vi "Remove Wall Complete Lines.vi"(8 "entrée d'erreur (pas d'erreur)":errorcluster, 9 "Lines Size List":i32[](array[numeric]), 10 "Brick Wall In":T1[](array[typedef]), 11 "Game Board In":refnum<class "Game Board.lvclass">) -> (0 "sortie d'erreur":errorcluster caption="error out", 1 "Brick Wall Out":T1[](array[typedef]), 3 "Game Board Out":refnum<class "Game Board.lvclass">)   [LabVIEW 2017, in "Game Board.lvclass"]
uses:
  Game Board.lvclass
  Controls/Coordinates.ctl
  Game Board.lvclass/Game Board.ctl
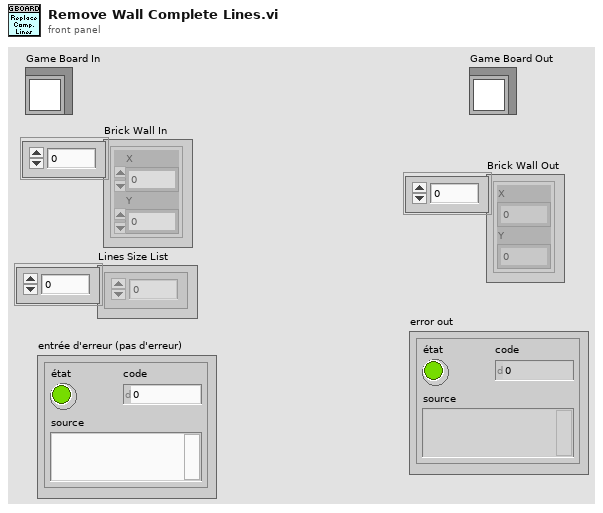
[diagram p1: front panel]
types:
  T1 = typedef "Coordinates.ctl" = cluster{"X":i32, "Y":i32}
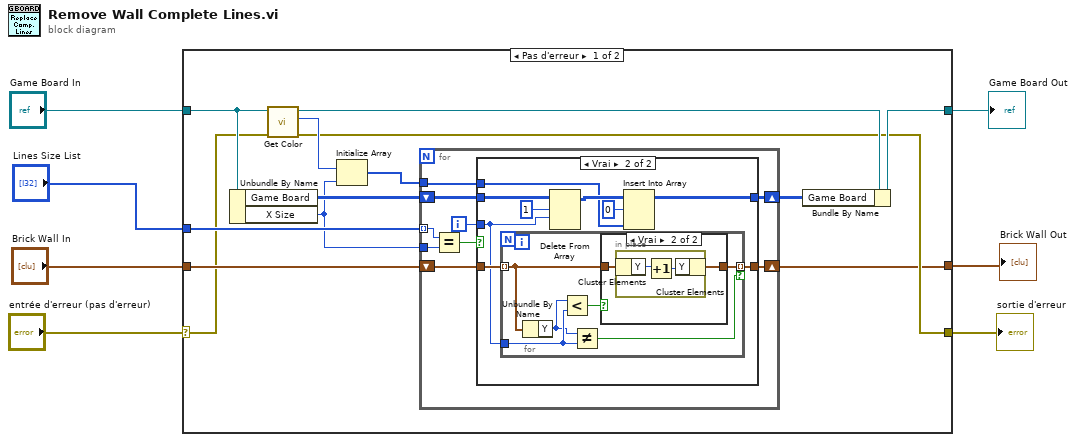
[diagram p0: block diagram]
diagram:
  n1 = case shown="Pas d'erreur" "entrée d'erreur (pas d'erreur)" {
    selector: "entrée d'erreur (pas d'erreur)" -> [w11 w53]
    tunnel: "Game Board In" -> [w12 w54]
    tunnel: [w10 w54] -> w5
    tunnel: [w9 w53] -> w4
    tunnel: "Brick Wall In" -> [w16 w52]
    tunnel: "Lines Size List" -> [w14 _]
    tunnel: [w8 w52] -> w1
    frame No Error {
      n2 = Unbundle By Name(w12) -> ("Game Board"=w17:u32[][], "X Size"=w13:i32)
      n3 = call-dynamic "Get Color.vi"("error in (no error)"=w11, "object in"=w12) -> ("error out"=w9:errorcluster, "Color"=w19:u32, "object out"=w18:refnum<class "Game Board.lvclass">)  [unwired: 7 in]
      n4 = Initialize Array(w19, w13) -> (w20:u32[])
      n5 = for {
        tunnel: w13 -> [w29]
        shift-right: [w27] -> w15
        shift-left: w17 -> [w28]
        tunnel: w20 -> [w24]
        shift-right: [w21] -> w8
        shift-left: w16 -> [w22]
        tunnel: w14 -> [w23] mode=indexing
        i -> [w25]
        n6 = Equal?(x=w23, y=w29) -> (x = y?=w26:bool)
        n7 = case shown="Vrai" w26 {
          tunnel: w28 -> [w31 w40]
          tunnel: [w31 w37] -> w27
          tunnel: w25 -> [_ w33]
          tunnel: w24 -> [_ w36]
          tunnel: w22 -> [w30 w35]
          tunnel: [w30 w34] -> w21
          frame False {
          }
          frame True {
            n8 = for {
              tunnel: w35 -> [w42] mode=indexing
              tunnel: [w41] -> w34 mode=indexing if=w46
              tunnel: w33 -> [w45]
              n9 = Unbundle By Name(w42) -> ("Y"=w44:i32)
              n10 = Less?(x=w44, y=w45) -> (x < y?=w43:bool)
              n11 = Not Equal?(x=w44, y=w45) -> (x != y?=w46:bool)
              n12 = case shown="Vrai" w43 {
                tunnel: w42 -> [w47 w49]
                tunnel: [w47 w48] -> w41
                frame False {
                }
                frame True {
                  n13 = in-place {
                    n14 = in-place-cluster #1(w49) -> ("Y"=w51:i32)
                    n15 = Increment(x=w51) -> (x+1=w50:i32)
                    n16 = in-place-cluster #1("Y"=w50) -> (w48:T1)
                  }
                }
              }
            }
            n17 = Delete From Array(array=w40, length=1 ("longueur"), index (row)=w33) -> (array with subset deleted=w38:u32[][])  [unwired: 1 in, 1 out]
            n18 = Insert Into Array(array=w38, index (row)=0 ("indice (ligne)"), new element=w36) -> (w37:u32[][])  [unwired: 1 in]
          }
        }
      }
      n19 = Bundle By Name(cluster=w18, "Game Board"=w15) -> (w10:refnum<class "Game Board.lvclass">)
    }
    frame Error {
    }
  }
  "Game Board Out" <- w5
  "sortie d'erreur" <- w4
  "Brick Wall Out" <- w1
